vi "Write Alarm Limits - High Warning Limit.vi"(8 "error in (no error)":errorcluster, 10 "high warning limit":dbl format="%.2f", 11 "NT Scalar (Numeric) in":refnum<class "NT Scalar (Numeric).lvclass">) -> (0 "error out":errorcluster, 3 "NT Scalar (Numeric) out":refnum<class "NT Scalar (Numeric).lvclass">)   [LabVIEW 2020, in "PV Access.lvlib" / "PV Data.lvlib" / "NT Scalar (Numeric).lvclass"]
uses:
  NT Scalar (Numeric).lvclass
  NT Scalar (Numeric).lvclass/NT Scalar (Numeric).ctl
  5b85e910-dd25-4407-becf-c3ddfd03cca0.vi
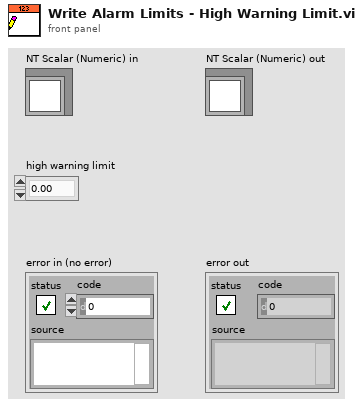
[diagram p1: front panel]
types:
  T1 = typedef "PV Access.lvlib/PV Data.lvlib/Type Code.ctl" = enum8{"Null", "Bool", "BoolA", "Int8", "Int8A", "Int16", "Int16A", "Int32", "Int32A", "Int64", "Int64A", "UInt8", "UInt8A", "UInt16", "UInt16A", "UInt32", "UInt32A", "UInt64", "UInt64A", "Float32", "Float32A", "Float64", "Float64A", "String", "StringA", "Struct", "StructA", "Union", "UnionA", "Any", "AnyA"}
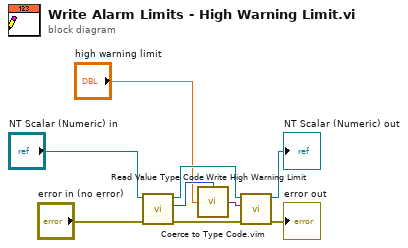
[diagram p0: block diagram]
diagram:
  n1 = call-dynamic "Read Value Type Code.vi"("error in (no error)"="error in (no error)", "NT Scalar in"="NT Scalar (Numeric) in") -> ("error out"=w6:errorcluster, "type code"=w7:T1, "NT Scalar out"=w3:refnum<class "NT Scalar (Numeric).lvclass">)  [unwired: 7 in]
  n2 = call "Coerce to Type Code.vim"("type code"=w7, "value in"="high warning limit") -> ("value out"=w1:variant)  [unwired: 2 in]
  n3 = call-dynamic "Write High Warning Limit.vi"("error in"=w6, "high warning limit"=w1, "Has Alarm Limits in"=w3) -> ("error out"=→"error out":errorcluster, "Has Alarm Limits out"=→"NT Scalar (Numeric) out":refnum<class "NT Scalar (Numeric).lvclass">)  [unwired: 7 in]
